vi "vision state ctrl.vi"(1 "Enable/Disable":bool) -> ()   [LabVIEW 2014]
uses:
  typedefs/vision/vision enable.ctl
  typedefs/vision/vision data.ctl
  vision.vi
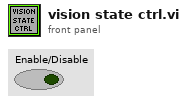
[diagram p1: front panel]
types:
  T1 = typedef "vision enable.ctl" = enum16{"Enable", "Disable", "Stop"}
  T2 = typedef "vision data.ctl" = cluster{"x":dbl, "y":dbl, "area":dbl, "width":dbl, "height":dbl}
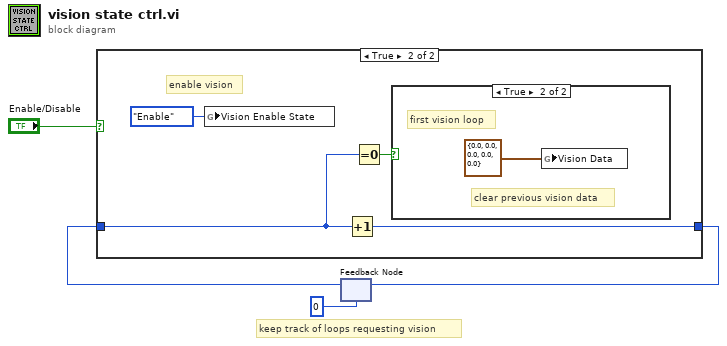
[diagram p0: block diagram]
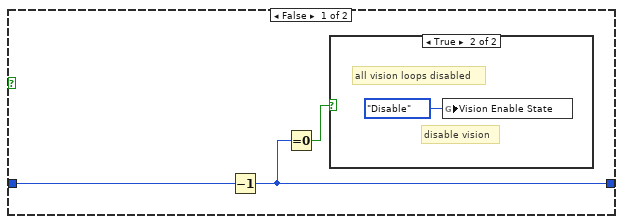
[diagram p2: hidden frame]
diagram:
  # "keep track of loops requesting vision"
  n1 = feedback #1(0) -> (w2:i32)
  n2 = case shown="True" "Enable/Disable" {
    tunnel: w2 -> [w7 w10]
    tunnel: [w6 w12] -> w1
    frame False {
      n3 = Decrement(x=w7) -> (x-1=w6:i32)
      n4 = Equal To 0?(x=w6) -> (x = 0?=w5:bool)
      n5 = case shown="True" w5 {
        frame False {
        }
        frame True {
          # "all vision loops disabled"
          # "disable vision"
          n6 = global write "vision.vi" "Vision Enable State"(vision_enable."Disable" ("Action")) -> ()
        }
      }
    }
    frame True {
      # "enable vision"
      n7 = global write "vision.vi" "Vision Enable State"(vision_enable."Enable" ("Action")) -> ()
      n8 = Increment(x=w10) -> (x+1=w12:i32)
      n9 = Equal To 0?(x=w10) -> (x = 0?=w11:bool)
      n10 = case shown="True" w11 {
        frame False {
          # "already enabled"
        }
        frame True {
          # "first vision loop"
          # "clear previous vision data"
          n11 = global write "vision.vi" "Vision Data"(T2 {"x"=0.0, "y"=0.0, "area"=0.0, "width"=0.0, "height"=0.0} ("Input")) -> ()
        }
      }
    }
  }
  n12 = feedback-in #1(w1) -> ()
